vi "NIIE_Selection_PrepareIcon.vi"(6 "Delete Selected Area?":bool, 8 "AntsRect":T1, 9 "AntsRect Orig":T1, 10 "new picture":picture, 11 "Layer.lvclass in":refnum<class "Layer.lvclass">) -> (3 "Layer.lvclass out":refnum<class "Layer.lvclass">)   [LabVIEW 2021]
uses:
  vi.lib/LabVIEW Icon API/lv_icon/Classes/Layer/Layer.lvclass
  vi.lib/LabVIEW Icon API/lv_icon/lv_icon.lvlib
panel:
  out "error out":errorcluster
  in  "error in (no error)":errorcluster
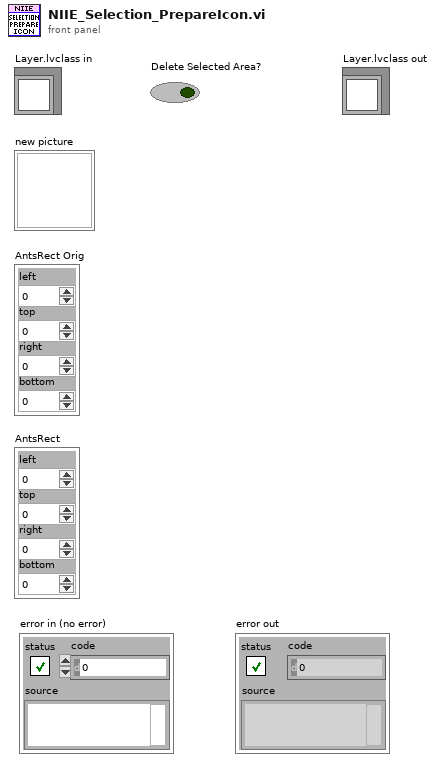
[diagram p1: front panel]
types:
  T1 = cluster{"left":i16, "top":i16, "right":i16, "bottom":i16}
  T2 = typedef "Cluster_Layer Data.ctl" = cluster{"LayerIcon":picture, "LayerName":string, "Opacity":u8, "Visibility?":bool}
  T3 = typedef "LVPositionTypeDef.ctl" = cluster{"Left":i32, "Top":i32}
  T4 = typedef "imagedata.ctl" = cluster{"image type":i32, "image depth":i32, "image":u8[], "mask":u8[], "colors":u32[], "Rectangle":cluster{"left":i16, "top":i16, "right":i16, "bottom":i16}}
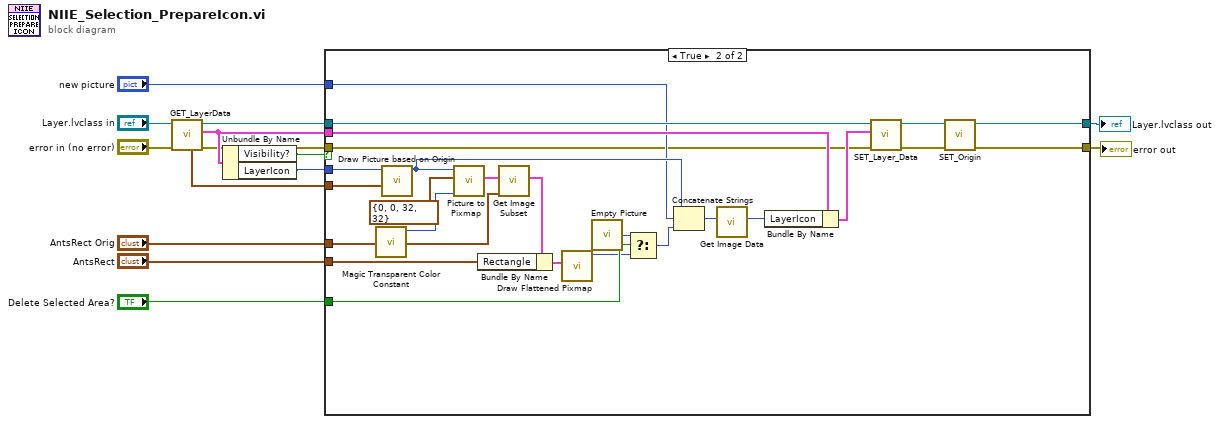
[diagram p0: block diagram]
diagram:
  n1 = call-dynamic "GET_LayerData.vi"("error in (no error)"="error in (no error)", "Layer.lvclass in"="Layer.lvclass in") -> ("error out"=w4:errorcluster, "Data"=w12:T2, "Layer.lvclass out"=w13:refnum<class "Layer.lvclass">, "Origin"=w8:T3)  [unwired: 6 out]
  n2 = Unbundle By Name(w12) -> ("Visibility?"=w1:bool, "LayerIcon"=w10:picture)
  n3 = case shown="True" w1 {
    tunnel: [w16 w18] -> w14
    tunnel: w13 -> [w16 w41]
    tunnel: w12 -> [_ w39]
    tunnel: "AntsRect" -> [_ w21]
    tunnel: w10 -> [_ w36]
    tunnel: "AntsRect Orig" -> [_ w35]
    tunnel: w8 -> [_ w22]
    tunnel: "Delete Selected Area?" -> [_ w29]
    tunnel: "new picture" -> [_ w28]
    tunnel: w4 -> [w15 w27]
    tunnel: [w15 w17] -> w2
    frame False {
    }
    frame True {
      n4 = call "Magic Transparent Color Constant.vi"() -> ("Magic transparent color constant"=w26:u32)  [unwired: 11 out]
      n5 = call "Draw Picture based on Origin.vi"("Origin"=w22, "LayerIcon in"=w36) -> ("LayerIcon out"=w32:picture)  [unwired: 1 in, 8 out]
      n6 = call <vilib>:"Picture to Pixmap.vi"("Background Color"=w26, "rect"=T1 {"left"=0, "top"=0, "right"=32, "bottom"=32}, "picture"=w32) -> ("image data"=w34:T4)  [unwired: 1 in, 7 out]
      n7 = call <vilib>:"Get Image Subset.vi"("subset rect"=w35, "image data"=w34) -> ("image subset"=w37:T4)  [unwired: 5 out]
      n8 = Bundle By Name(cluster=w37, "Rectangle"=w21) -> (w38:T4)
      n9 = call <vilib>:"Draw Flattened Pixmap.vi"("image data"=w38) -> ("new picture"=w25:picture)  [unwired: 1 in, 7 out]
      n10 = call "Empty Picture"() -> ("empty picture"=w30:picture)
      n11 = Select(t=w30, s=w29, f=w25) -> (s? t:f=w31:picture)
      n12 = Concatenate Strings(w32, w28, w31) -> (w24:picture)
      n13 = call "Get Image Data.vi"("Pic"=w24) -> ("Pic Out"=w23:picture)  [unwired: 1 in, 9 out]
      n14 = Bundle By Name(cluster=w39, "LayerIcon"=w23) -> (w40:T2)
      n15 = call-dynamic "SET_Layer_Data.vi"("error in (no error)"=w27, "Data"=w40, "Layer.lvclass in"=w41) -> ("error out"=w20:errorcluster, "Layer.lvclass out"=w19:refnum<class "Layer.lvclass">)  [unwired: 1 in, 6 out]
      n16 = call-dynamic "SET_Origin.vi"("error in (no error)"=w20, "Layer.lvclass in"=w19) -> ("error out"=w17:errorcluster, "Layer.lvclass out"=w18:refnum<class "Layer.lvclass">)  [unwired: 8 in]
    }
  }
  "Layer.lvclass out" <- w14
  "error out" <- w2
